vi "Auton File Read.vi"(8 "error in (no error)":errorcluster, 11 "Script Path":string) -> (0 "error out":errorcluster, 1 "New Script Loaded":bool, 3 "Auton Parameters":T1)   [LabVIEW 2015]
panel:
  out "Parameter Values":dbl[](array[numeric])
  out "Parameter Type":string[](array[string])
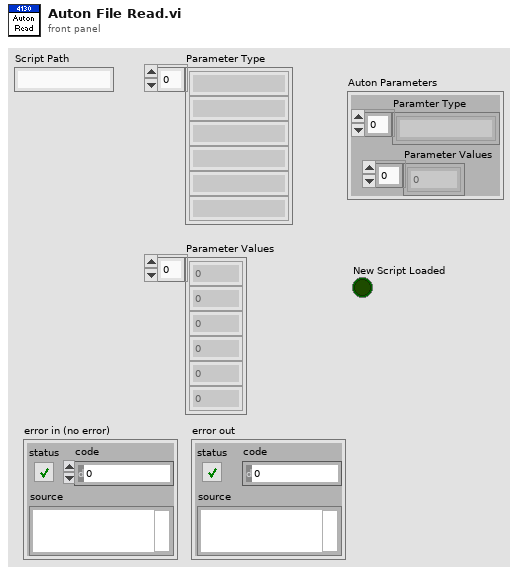
[diagram p1: front panel]
types:
  T1 = cluster{"Paramter Type":string[], "Parameter Values":dbl[]}
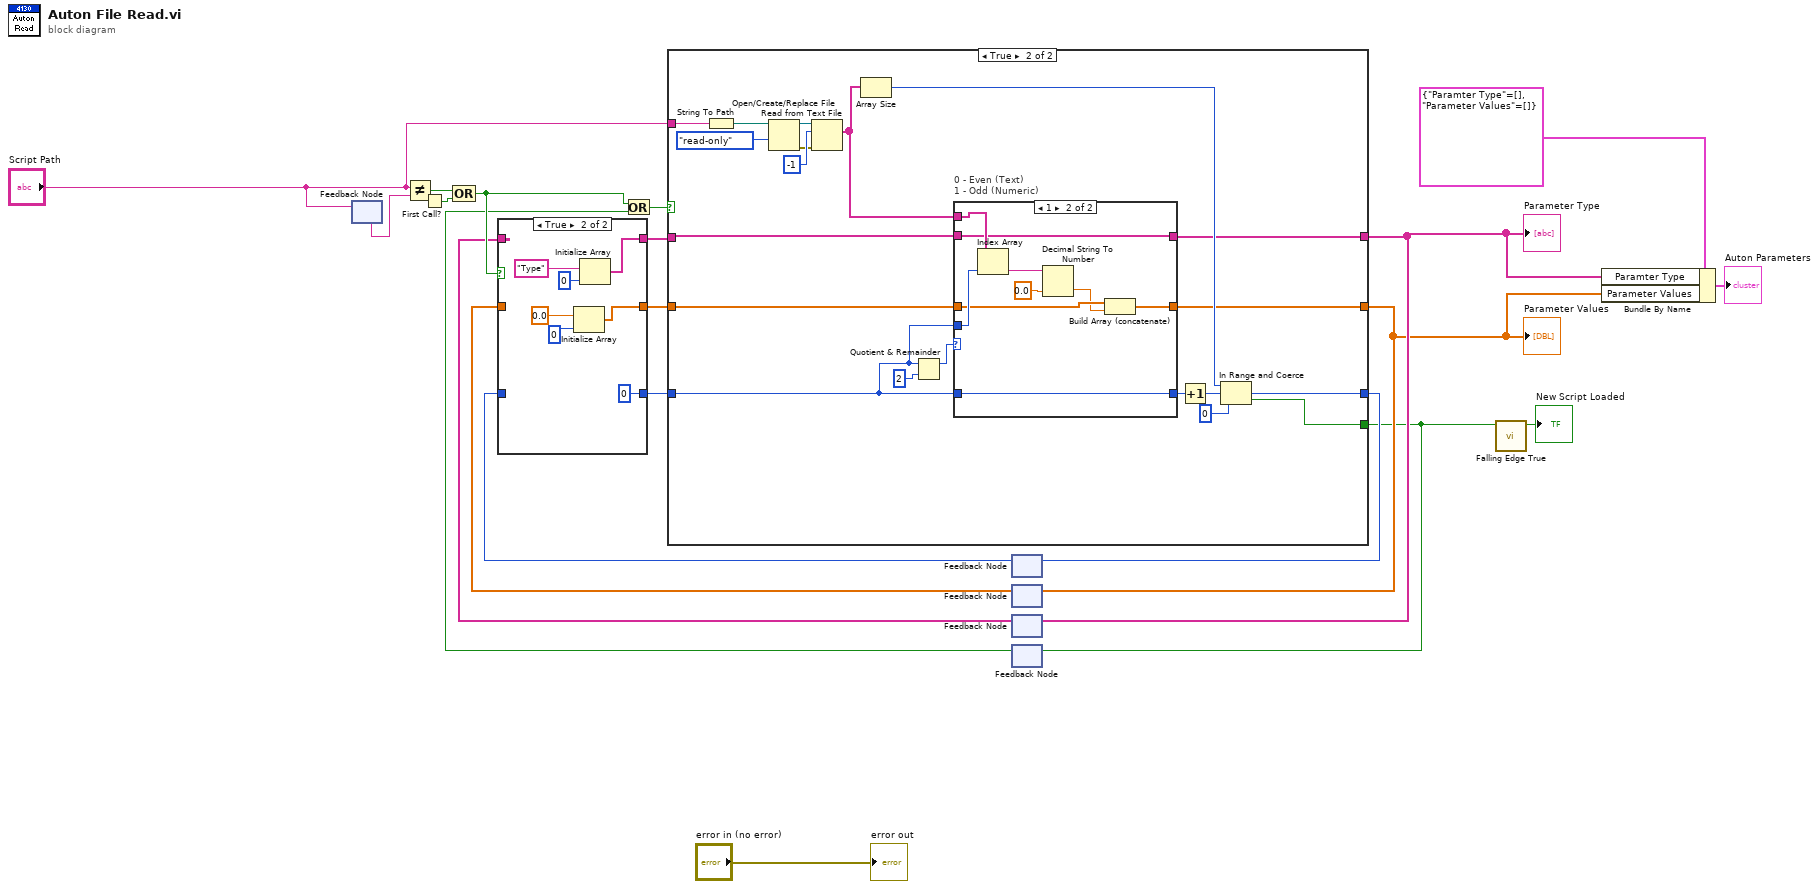
[diagram p0: block diagram]
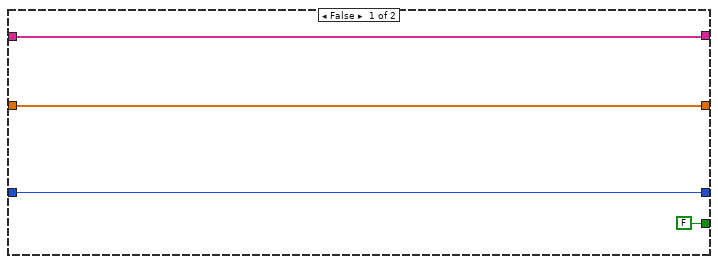
[diagram p3: hidden frame]
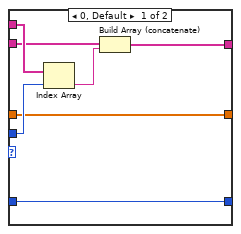
[diagram p4: hidden frame]
diagram:
  n1 = feedback #1() -> (w8:string)  [unwired: 1 in]
  n2 = feedback-in #1("Script Path") -> ()
  n3 = Not Equal?(x="Script Path", y=w8) -> (x != y?=w12:bool)
  n4 = First Call?() -> (First Call?: T/F=w13:bool)
  n5 = Compound Arithmetic op=OR(w12, w13) -> (w18:bool)
  n6 = feedback #2() -> (w20:i32)  [unwired: 1 in]
  n7 = feedback #3() -> (w16:dbl[])  [unwired: 1 in]
  n8 = feedback #4() -> (w14:string[])  [unwired: 1 in]
  n9 = case shown="True" w18 {
    tunnel: w14 -> [w24 _]
    tunnel: [w24 w29] -> w15
    tunnel: w16 -> [w23 _]
    tunnel: [w23 w26] -> w17
    tunnel: w20 -> [w22 _]
    tunnel: [w22 0 ("lower limit")] -> w21
    frame False {
    }
    frame True {
      n10 = Initialize Array(0.0, 0 ("dimension size")) -> (w26:dbl[])
      n11 = Initialize Array("Type" ("string"), 0 ("dimension size")) -> (w29:string[])
    }
  }
  n12 = feedback #5() -> (w11:bool)  [unwired: 1 in]
  n13 = Or(x=w18, y=w11) -> (x .or. y?=w10:bool)
  n14 = case shown="True" w10 {
    tunnel: "Script Path" -> [_ w54]
    tunnel: [w35 w42] -> w6
    tunnel: [w34 w41] -> w5
    tunnel: w15 -> [w35 w39]
    tunnel: w17 -> [w34 w38]
    tunnel: [FALSE w40] -> w3
    tunnel: [w32 w37] -> w19
    tunnel: w21 -> [w32 w36]
    frame False {
    }
    frame True {
      n15 = String To Path(string=w54) -> (path=w55:path)
      n16 = Open/Create/Replace File(file path (use dialog)=w55, access (0:read/write)=enum16{"read/write", "read-only", "write-only"}."read-only") -> (refnum out=w51:refnum<file>, error out=w50:errorcluster)  [unwired: 4 in, 1 out]
      n17 = Read from Text File(file (use dialog)=w51, count=-1, error in=w50) -> (text=w43:string[])  [unwired: 1 in, 3 out]
      n18 = Array Size(array=w43) -> (size(s)=w46:i32)
      n19 = Quotient & Remainder(x=w36, y=2) -> (x-y*floor(x/y)=w44:i32)  [unwired: 1 out]
      n20 = case "0 - Even (Text)\n1 - Odd (Numeric)" shown="1" w44 {
        tunnel: w36 -> [w62 w71]
        tunnel: [w62 w71] -> w49
        tunnel: w39 -> [w58 w65]
        tunnel: w38 -> [w56 w64]
        tunnel: w36 -> [w60 w69]
        tunnel: w43 -> [w61 w70]
        tunnel: [w57 w65] -> w42
        tunnel: [w56 w66] -> w41
        frame 0, Default {
          n21 = Index Array(array=w61, index=w60) -> (element=w59:string)
          n22 = Build Array (concatenate)(w58, w59) -> (w57:string[])
        }
        frame 1 {
          n23 = Index Array(array=w70, index=w69) -> (element=w68:string)
          n24 = Decimal String To Number(string=w68, default (0L)=0.0) -> (number=w63:dbl)  [unwired: 1 in, 1 out]
          n25 = Build Array (concatenate)(w64, w63) -> (w66:dbl[])
        }
      }
      n26 = Increment(x=w49) -> (x+1=w48:i32)
      n27 = In Range and Coerce(upper limit=w46, x=w48, lower limit=0) -> (coerced(x)=w37:i32, In Range?=w40:bool)
    }
  }
  "Parameter Type" <- w6
  "Parameter Values" <- w5
  n28 = feedback-in #2(w19) -> ()
  n29 = feedback-in #3(w5) -> ()
  n30 = feedback-in #4(w6) -> ()
  n31 = feedback-in #5(w3) -> ()
  n32 = call "Falling Edge True.vi"("Input"=w3) -> ("Output"=→"New Script Loaded":bool)  [unwired: 10 in]
  n33 = Bundle By Name(cluster=T1 {"Paramter Type"=[], "Parameter Values"=[]}, "Paramter Type"=w6, "Parameter Values"=w5) -> (→"Auton Parameters":T1)
  "error out" <- "error in (no error)"
